vi "Parse String.vi"(4 "dst byte order":T1(ring), 6 "src byte order":T1(ring), 7 "conversions":T2[](array[typedef]) {"converted descriptor"."buffer offset" format="%d bytes"; "unconverted descriptor"."buffer offset" format="%d bytes"}, 8 "error in (no error)":errorcluster, 9 "dst buffer in":string, 10 "src buffer in":string, 11 "Buffer Converter in":refnum<class "Buffer Converter.lvclass">) -> (0 "error out":errorcluster, 1 "dst buffer out":string, 2 "src buffer out":string, 3 "Buffer Converter out":refnum<class "Buffer Converter.lvclass">)   [LabVIEW 2017, in "DSF Core.lvlib" / "Buffer Converter.lvclass"]
uses:
  Buffer Converter.lvclass
  Conversion.ctl
  Block Descriptor.ctl
  DSF Configuration API/Public/Controls/DSF Data Type.ctl
  DSF Core.lvlib
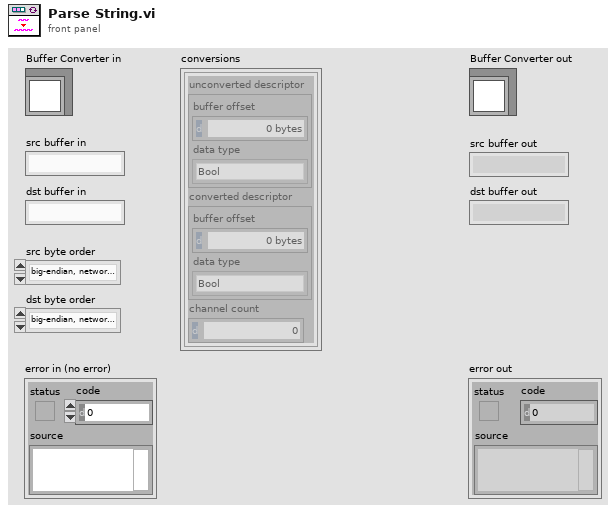
[diagram p1: front panel]
types:
  T1 = enum16{"big-endian, network order", "native, host order", "little-endian"}
  T2 = typedef "DSF Core.lvlib/Buffer Converter.lvclass/Conversion.ctl" = cluster{"unconverted descriptor":T3, "converted descriptor":T3, "channel count":u64}
  T3 = typedef "DSF Core.lvlib/Buffer Converter.lvclass/Block Descriptor.ctl" = cluster{"buffer offset":u64, "data type":T4}
  T4 = typedef "DSF Core.lvlib/DSF Data Type.ctl" = enum8{"Bool", "SGL", "DBL", "I8", "I16", "I32", "I64", "U8", "U16", "U32", "U64"}
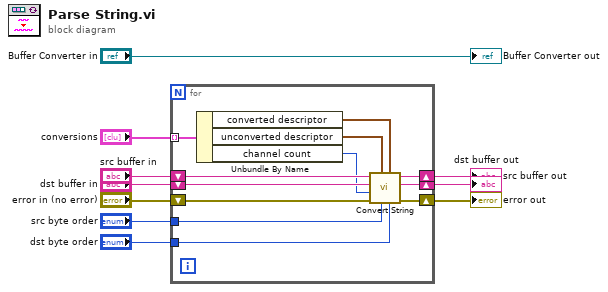
[diagram p0: block diagram]
diagram:
  n1 = for {
    shift-right: [w17] -> w3
    shift-left: "error in (no error)" -> [w22]
    shift-right: [w18] -> w4
    shift-left: "dst buffer in" -> [w21]
    shift-right: [w20] -> w2
    shift-left: "src buffer in" -> [w19]
    tunnel: "src byte order" -> [w16]
    tunnel: "dst byte order" -> [w15]
    tunnel: "conversions" -> [w14] mode=indexing
    n2 = Unbundle By Name(w14) -> ("converted descriptor"=w12:T3, "unconverted descriptor"=w13:T3, "channel count"=w11:u64)
    n3 = call "Convert String.vi"("dst byte order"=w15, "src channel descriptor"=w12, "src byte order"=w16, "dst channel descriptor"=w13, "error in (no error)"=w22, "channel count"=w11, "dst buffer in"=w21, "src buffer in"=w19) -> ("error out"=w17:errorcluster, "dst buffer out"=w18:string, "src buffer out"=w20:string)  [unwired: 1 in]
  }
  "error out" <- w3
  "dst buffer out" <- w4
  "src buffer out" <- w2
  "Buffer Converter out" <- "Buffer Converter in"
